vi "PopulateTest.vi"() -> (0 "error out":errorcluster, 2 "Pass":bool)   [LabVIEW 2025, in "NISE_CEF_Tests.lvlib"]
uses:
  NISE_CEF_Tests.lvlib
panel:
  out "All Tags":string[](array[string])
  in  "View":string(tree)
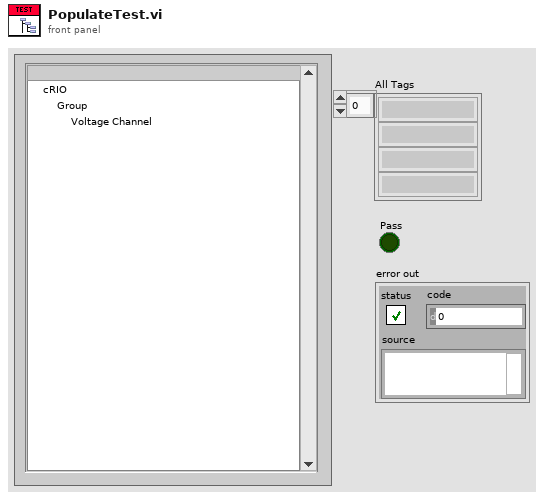
[diagram p1: front panel]
types:
  T1 = typedef "NISE_CEF_Node.lvclass/Summary.ctl" = cluster{"ID":string, "parent ID":string, "node type":string, "text":string, "additional text":string, "glyph":string, "depth":i32, "glyph overlay":string}
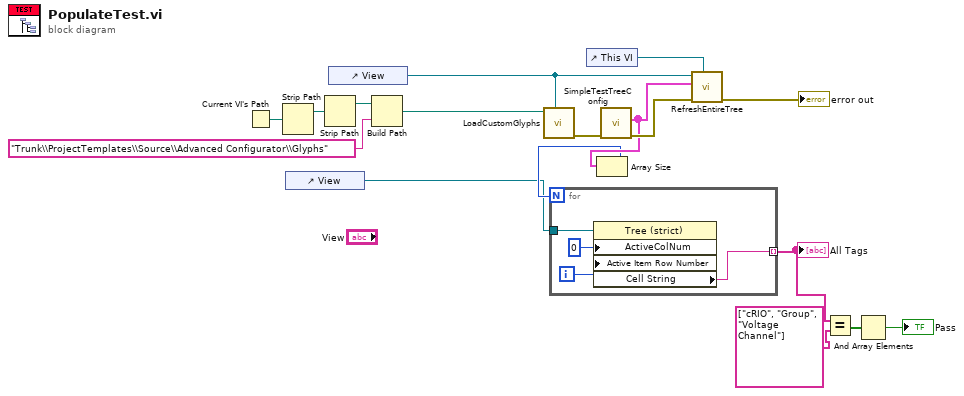
[diagram p0: block diagram]
diagram:
  n1 = Current VI's Path() -> (path=w12:path)
  n2 = Strip Path(path=w12) -> (stripped path=w11:path)  [unwired: 1 out]
  n3 = control-ref of="View"() -> (w5:refnum<vi>)
  n4 = Strip Path(path=w11) -> (stripped path=w10:path)  [unwired: 1 out]
  n5 = control-ref of="View"() -> (w17:refnum<vi>)
  n6 = Build Path(base path=w10, name or relative path="Trunk\\ProjectTemplates\\Source\\Advanced Configurator\\Glyphs") -> (appended path=w8:path)
  n7 = call "LoadCustomGlyphs.vi"("tree ref"=w17, "glyph directory"=w8) -> ("error out"=w14:errorcluster)  [unwired: 9 in]
  n8 = control-ref of="This VI"() -> (w16:refnum<vi>)
  n9 = call "SimpleTestTreeConfig.vi"("error in"=w14) -> ("error out"=w13:errorcluster, "summary"=w7:T1[])  [unwired: 8 in, 1 out]
  n10 = Array Size(array=w7) -> (size(s)=w6:i32)
  n11 = for {
    N: w6 -> [_]
    tunnel: [w18] -> w3 mode=indexing
    tunnel: w5 -> [w21]
    i -> [w20]
    n12 = property class="Tree (strict)"(reference=w21, "ActiveColNum"=0 ("Active Cell:Active Column Number"), "Active Item Row Number"=w20) -> ("Cell String"=w18:string)  [unwired: 1 in, 2 out]
  }
  "All Tags" <- w3
  n13 = call "RefreshEntireTree.vi"("calling VI in"=w16, "error in"=w13, "array"=w7, "tree ref in"=w17) -> ("error out"=→"error out":errorcluster)  [unwired: 7 in]
  n14 = Equal?(x=w3, y=string[] ["cRIO", "Group", "Voltage Channel"] ("All Tags")) -> (x = y?=w2:bool[])
  n15 = And Array Elements(Boolean array=w2) -> (logical AND=→"Pass":bool)
